vi "TriggerTests_2_clip.vi"() -> ()   [LabVIEW 2009]
uses:
  <vilib>/Utility/NIReport.llb/NI_report.lvclass
  <instrlib>/Agilent 81150/Agilent 81150.lvlib
panel:
  in  "error in":errorcluster
  out "50%":dbl[][][][](array[numeric])
  in  "Init att value":i32[](array[numeric])
  in  "Init clip value":i32[](array[numeric])
  in  "Voltages values":dbl[](array[numeric])
  in  "nm ch":i32[](array[numeric])
  in  "Instrument VISA in":T1={"AWG VISA"="81160A", "Oscilloscope  VISA "="DSO80204B", "Integration Board IP"="172.16.7.43", "connection ID"=refnum, "report out"=refnum, "report file path"=path "D:/CTA/LevelTriggerBoardTest/TestsData/sumtrigger_delay"}
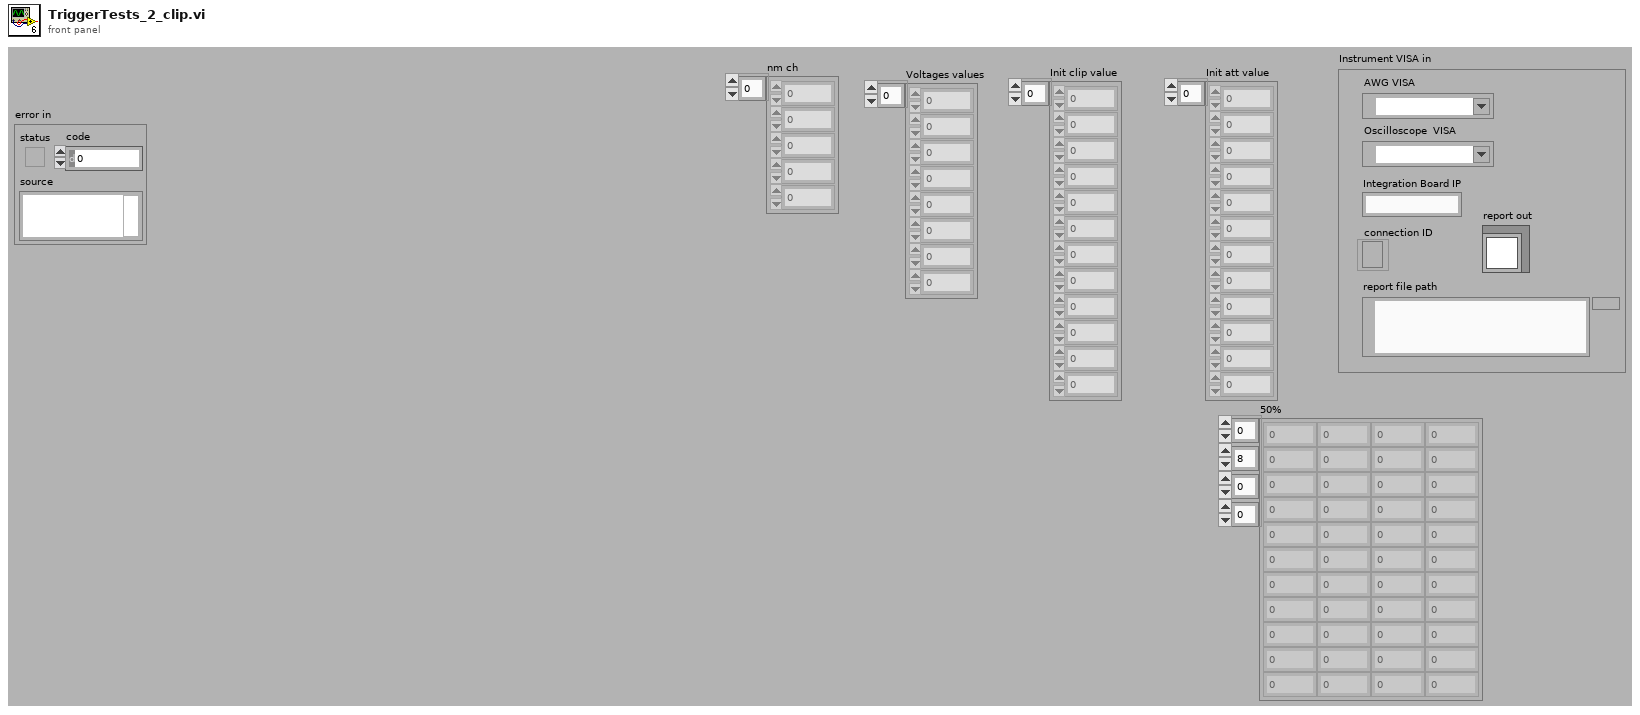
[diagram p1: front panel]
types:
  T1 = cluster{"AWG VISA":refnum<visa-resource-name>, "Oscilloscope  VISA ":refnum<visa-resource-name>, "Integration Board IP":string, "connection ID":refnum<k5>, "report out":refnum<class "NI_report.lvclass">, "report file path":path}
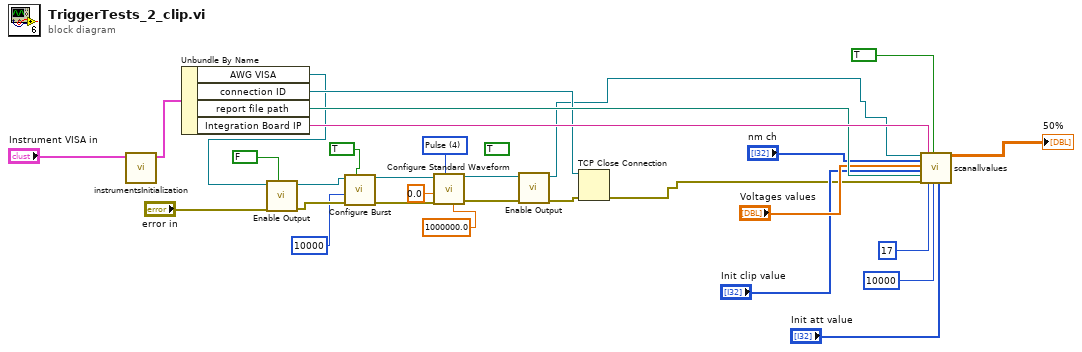
[diagram p0: block diagram]
diagram:
  (unwired) TRUE ("Enable Output (T: Enable)")
  w16 = u16 4 items=["Sine", "Square", "Ramp Up", "Ramp Down", "Pulse", "Noise", "DC"] ("Waveform (0: Sine)")
  n1 = call "instrumentsInitialization.vi"("Instrument VISA in"="Instrument VISA in") -> ("Instrument VISA out"=w26:T1)  [unwired: 9 in, 1 out]
  n2 = Unbundle By Name(w26) -> ("AWG VISA"=w2:refnum<visa-resource-name>, "connection ID"=w6:refnum<k5>, "report file path"=w24:path, "Integration Board IP"=w25:string)
  n3 = call <instrlib>:"Enable Output.vi"("Enable Output (T: Enable)"=FALSE, "error in (no error)"="error in", "VISA resource name"=w2) -> ("error out"=w9:errorcluster, "VISA resource name out"=w8:refnum<visa-resource-name>)  [unwired: 7 in]
  n4 = call <instrlib>:"Configure Burst.vi"("Enable Burst (F: Disable)"=TRUE, "error in (no error)"=w9, "Burst Count (2)"=10000, "VISA resource name"=w8) -> ("error out"=w14:errorcluster, "VISA resource name out"=w15:refnum<visa-resource-name>)  [unwired: 6 in]
  n5 = call <instrlib>:"Configure Standard Waveform.vi"("Frequency (1000.0 Hz)"=1000000.0, "Waveform (0: Sine)"=w16, "error in (no error)"=w14, "Amplitude (1.0 Vpp)"=0.0, "VISA resource name"=w15) -> ("error out"=w13:errorcluster, "VISA resource name out"=w12:refnum<visa-resource-name>)  [unwired: 5 in]
  n6 = call <instrlib>:"Enable Output.vi"("error in (no error)"=w13, "VISA resource name"=w12) -> ("error out"=w10:errorcluster, "VISA resource name out"=w1:refnum<visa-resource-name>)  [unwired: 8 in]
  n7 = TCP Close Connection(connection ID=w6, error in (no error)=w10) -> (error out=w7:errorcluster)  [unwired: 1 in, 1 out]
  n8 = call "scanallvalues.vi"("VISA resource name out"=w1, "nm ch"="nm ch", "Voltages values"="Voltages values", "Init clip value"="Init clip value", "base path"=w24, "error in"=w7, "Integration Board IP"=w25, "L1 Address"=17, "Save test data"=TRUE ("Report Enable"), "Ch burst"=10000, "Init att value"="Init att value") -> ("50%"=→"50%":dbl[][][][])  [unwired: 6 in, 2 out]
